vi "Cal Plot Scale.vi"(8 "error in (no error)":errorcluster, 11 "Domain_Evolut_2D_Rect in":refnum<class "NI_Domain_Evolut_2D_Rect.lvclass">) -> (0 "error out":errorcluster, 1 "Y Scale":T1, 2 "X Scale":T1, 3 "Domain_Evolut_2D_Rect out":refnum<class "NI_Domain_Evolut_2D_Rect.lvclass">, 4 "# of t-points":i32)   [LabVIEW 2020, in "NI_PDE.lvlib" / "NI_Domain_Evolut_2D_Rect.lvclass"]
uses:
  <vilib>/gmath/pde.llb/DomainClass/Domain_Evolut_2D_Rect/NI_Domain_Evolut_2D_Rect.lvclass
  <vilib>/Utility/miscctls.llb/LVOffsetAndMultiplierTypeDef.ctl
  <vilib>/gmath/pde.llb/DomainClass/Domain_Evolut_2D_Rect/NI_Domain_Evolut_2D_Rect.lvclass/NI_Domain_Evolut_2D_Rect.ctl
  <vilib>/gmath/NI_PDE.lvlib
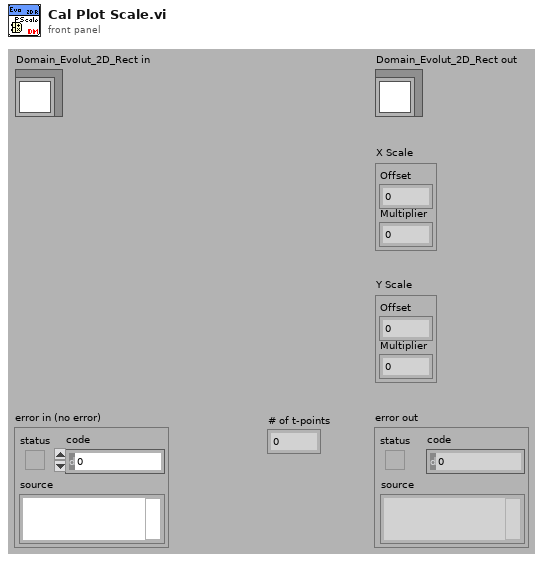
[diagram p1: front panel]
types:
  T1 = typedef "LVOffsetAndMultiplierTypeDef.ctl" = cluster{"Offset":dbl, "Multiplier":dbl}
  T2 = cluster{"initial t":dbl, "final t":dbl, "# of t-points":i32}
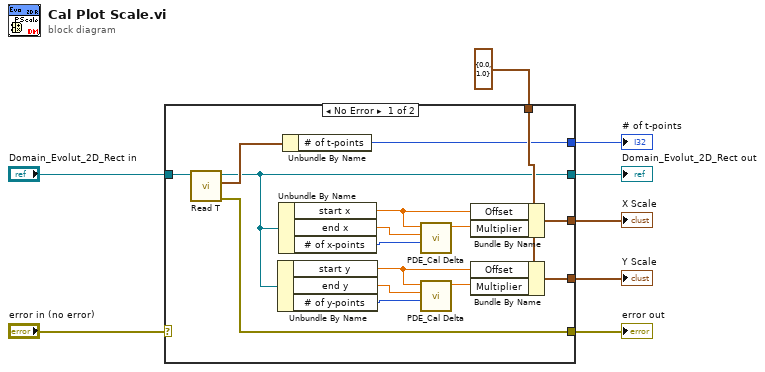
[diagram p0: block diagram]
diagram:
  n1 = case shown="No Error" "error in (no error)" {
    selector: "error in (no error)" -> [_ w27]
    tunnel: "Domain_Evolut_2D_Rect in" -> [w24 w26]
    tunnel: [w9 w26] -> w8
    tunnel: [w23 w27] -> w7
    tunnel: T1 {"Offset"=0.0, "Multiplier"=1.0} ("Offset and Multiplier") -> [w14 w25]
    tunnel: [w13 w25] -> w3
    tunnel: [w12 w25] -> w2
    tunnel: [w10 _] -> w1
    frame No Error {
      n2 = call-dynamic "Read T.vi"("Domain_Evolut.lvclass in"=w24) -> ("error out"=w23:errorcluster, "t"=w11:T2, "Domain_Evolut.lvclass out"=w9:refnum<class "NI_Domain_Evolut_2D_Rect.lvclass">)  [unwired: 1 in, 7 out]
      n3 = Unbundle By Name(w9) -> ("start y"=w16:dbl, "end y"=w18:dbl, "# of y-points"=w17:i32)
      n4 = Unbundle By Name(w9) -> ("start x"=w21:dbl, "end x"=w19:dbl, "# of x-points"=w20:i32)
      n5 = Unbundle By Name(w11) -> ("# of t-points"=w10:i32)
      n6 = call <vilib>:"PDE_Cal Delta.vi"("# of points"=w20, "end"=w19, "start"=w21) -> ("delta"=w22:dbl)  [unwired: 8 out]
      n7 = call <vilib>:"PDE_Cal Delta.vi"("# of points"=w17, "end"=w18, "start"=w16) -> ("delta"=w15:dbl)  [unwired: 8 out]
      n8 = Bundle By Name(cluster=w14, "Offset"=w21, "Multiplier"=w22) -> (w13:T1)
      n9 = Bundle By Name(cluster=w14, "Offset"=w16, "Multiplier"=w15) -> (w12:T1)
    }
    frame Error {
    }
  }
  "Domain_Evolut_2D_Rect out" <- w8
  "error out" <- w7
  "X Scale" <- w3
  "Y Scale" <- w2
  "# of t-points" <- w1
